vi "TX ADU.vi"(8 "error in (no error)":errorcluster, 9 "PDU_req in":T1={"Function Code"=1, "Data"=[], "RTU_DataBytes"=0}, 10 "TCP connection in":refnum<k5>, 11 "MB_ADU_TCP in":refnum<class "MB_ADU_TCP.lvclass">) -> (0 "error out":errorcluster, 1 "PDU_req out":T1={"Function Code"=1, "Data"=[], "RTU_DataBytes"=0}, 2 "TCP connection out":refnum<k5>, 3 "MB_ADU_TCP out":refnum<class "MB_ADU_TCP.lvclass">)   [LabVIEW 2012, in "MB Master.lvlib" / "MB_ADU_TCP.lvclass"]
doc: "Defines the transmit procedure for a Modbus TCP ADU. The PDU to be transmitted should be written to PDU_req prior to calling this VI."
uses:
  MB_ADU_TCP.lvclass
  MB_PDU/MB_PDU_Cluster.ctl
  MB_ADU_TCP.lvclass/MB_ADU_TCP.ctl
  MB_ADU/MB_ADU.lvclass/MB_ADU.ctl
  MB_ADU/Read Slave ID.vi
  MB_ADU/Write TX Data.vi
  MB_ADU/Write TX Timestamp.vi
  MB Master.lvlib
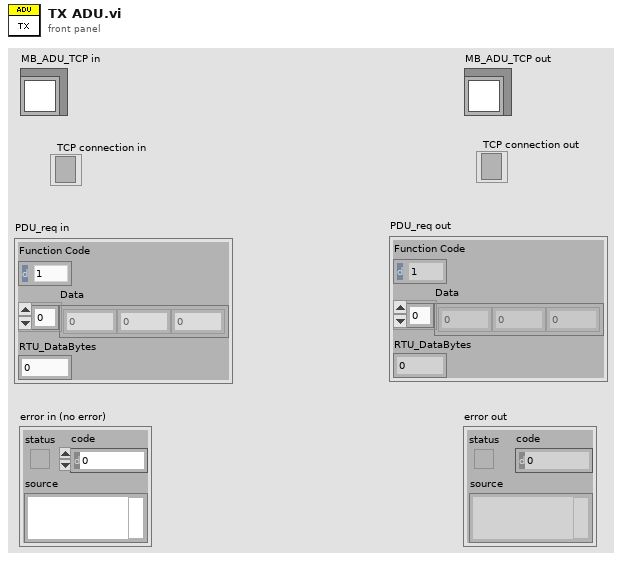
[diagram p1: front panel]
types:
  T1 = typedef "MB Master.lvlib/MB_PDU_Cluster.ctl" = cluster{"Function Code":u8, "Data":u8[], "RTU_DataBytes":i32}
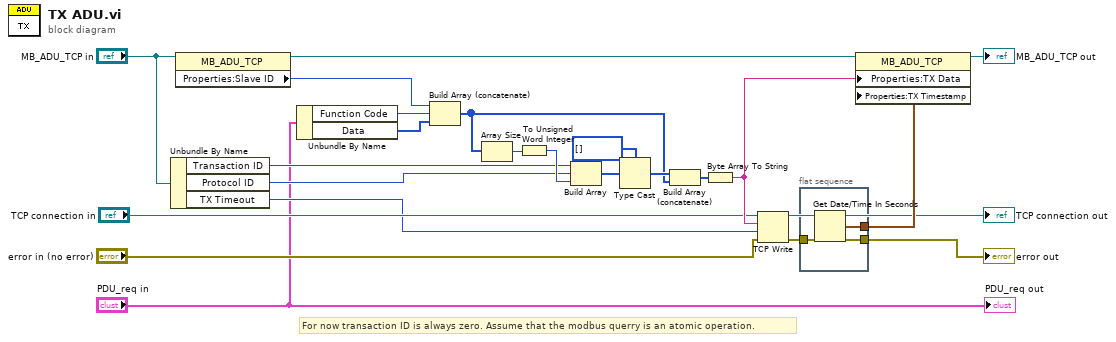
[diagram p0: block diagram]
diagram:
  # "For now transaction ID is always zero. Assume that the modbus querry is an atomic operation."
  n1 = Unbundle By Name("MB_ADU_TCP in") -> ("Transaction ID"=w11:u16, "Protocol ID"=w10:u16, "TX Timeout"=w4:i32)
  n2 = property class="MB_ADU_TCP"(reference="MB_ADU_TCP in") -> (reference out=w24:refnum<class "MB_ADU_TCP.lvclass">, "Properties:Slave ID"=w22:u8)  [unwired: 1 in, 1 out]
  n3 = Unbundle By Name("PDU_req in") -> ("Function Code"=w3:u8, "Data"=w2:u8[])
  n4 = Build Array (concatenate)(w22, w3, w2) -> (w16:u8[])
  n5 = Array Size(array=w16) -> (size(s)=w21:i32)
  n6 = To Unsigned Word Integer(number=w21) -> (unsigned 16bit integer=w20:u16)
  n7 = Build Array(w11, w10, w20) -> (w19:u16[])
  n8 = Type Cast(type=u8[] [], x=w19) -> (*(type *) &x=w17:u8[])
  n9 = Build Array (concatenate)(w17, w16) -> (w15:u8[])
  n10 = Byte Array To String(unsigned byte array=w15) -> (string=w8:string)
  n11 = TCP Write(connection ID="TCP connection in", data in=w8, error in (no error)="error in (no error)", 9:w4) -> (connection ID out=→"TCP connection out":refnum<k5>, error out=w9:errorcluster)  [unwired: 1 out]
  n12 = flat-sequence {
    tunnel: w9 -> [w26]
    tunnel: [w26] -> w14
    tunnel: [w25] -> w13
    frame #0 {
      n13 = Get Date/Time In Seconds() -> (seconds since 1Jan1904=w25:timestamp)
    }
  }
  n14 = property class="MB_ADU_TCP"(reference=w24, "Properties:TX Data"=w8, "Properties:TX Timestamp"=w13) -> (reference out=→"MB_ADU_TCP out":refnum<class "MB_ADU_TCP.lvclass">)  [unwired: 1 in, 1 out]
  "error out" <- w14
  "PDU_req out" <- "PDU_req in"
